vi "Enqueue User Que with Error Support.vi"(7 "コマンド":string, 8 "エラー入力（エラーなし）":errorcluster, 9 "タイムアウト（ms）（-1）":i32=-1, 10 "バリアント":variant, 11 "queVariant":refnum<queue>) -> (0 "エラー出力":errorcluster, 1 "timeout/overflow?":bool, 3 "queVariant(copy)":refnum<queue>)   [LabVIEW 2014]
uses:
  QueData.ctl
panel:
  in  "モード(Normal)":enum16{"Normal", "Lossy", "OppositeEnd"}(ring)
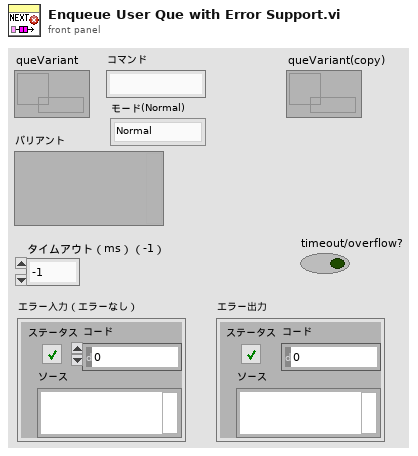
[diagram p1: front panel]
types:
  T1 = typedef "QueData.ctl" = cluster{"コマンド":string, "バリアント":variant}
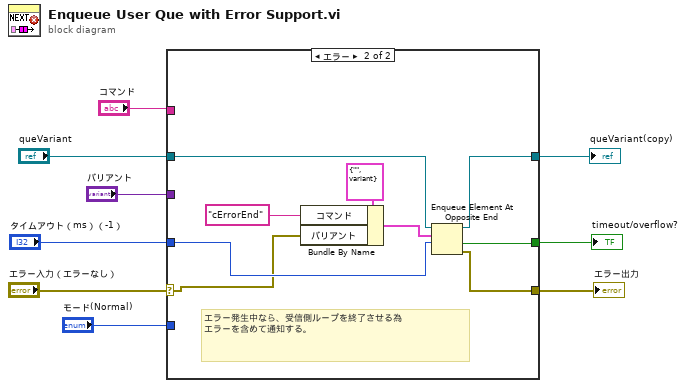
[diagram p0: block diagram]
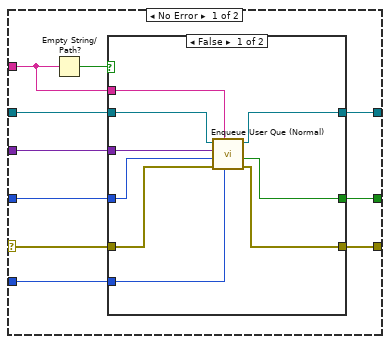
[diagram p2: hidden frame]
diagram:
  n1 = case shown="エラー" "エラー入力（エラーなし）" {
    selector: "エラー入力（エラーなし）" -> [w16 w32]
    tunnel: "queVariant" -> [w18 w34]
    tunnel: [w17 w35] -> w8
    tunnel: [w15 w31] -> w6
    tunnel: [w13 w37] -> w5
    tunnel: "タイムアウト（ms）（-1）" -> [w14 w36]
    tunnel: "コマンド" -> [w12 _]
    tunnel: "バリアント" -> [w11 _]
    tunnel: "モード(Normal)" -> [w10 _]
    frame No Error {
      n2 = Empty String/Path?(string/path=w12) -> (empty?=w19:bool)
      n3 = case shown="FALSE" w19 {
        tunnel: w18 -> [w28 w30]
        tunnel: [w21 w30] -> w17
        tunnel: w16 -> [w24 w29]
        tunnel: [w23 w29] -> w15
        tunnel: w11 -> [w26 _]
        tunnel: w14 -> [w25 _]
        tunnel: w12 -> [w27 _]
        tunnel: [w20 _] -> w13
        tunnel: w10 -> [w22 _]
        frame False {
          n4 = call "Enqueue User Que (Normal).vi"("モード(Normal)"=w22, "コマンド"=w27, "エラー入力（エラーなし）"=w24, "タイムアウト（ms）（-1）"=w25, "バリアント"=w26, "queVariant"=w28) -> ("エラー出力"=w23:errorcluster, "timeout/overflow?"=w20:bool, "queVariant(copy)"=w21:refnum<queue>)  [unwired: 3 in]
        }
        frame True {
        }
      }
    }
    frame Error {
      # "エラー発生中なら、受信側ループを終了させる為\nエラーを含めて通知する。"
      n5 = Bundle By Name(cluster=T1 {"コマンド"="", "バリアント"=variant} ("要素"), "コマンド"="cErrorEnd", "バリアント"=w32) -> (w38:T1)
      n6 = Enqueue Element At Opposite End(queue=w34, element=w38, timeout in ms (-1)=w36) -> (queue out=w35:refnum<queue>, timed out?=w37:bool, error out=w31:errorcluster)  [unwired: 1 in]
    }
  }
  "エラー出力" <- w6
  "queVariant(copy)" <- w8
  "timeout/overflow?" <- w5
